vi "Request Config Info.vi"(8 "error in (no error)":errorcluster, 11 "Config Monitor Module in":refnum<class "Config Monitor Module.lvclass">) -> (0 "error out":errorcluster, 3 "Config Monitor Module out":refnum<class "Config Monitor Module.lvclass">)   [LabVIEW 2020, in "VolatusGUI.lvlib" / "Config Monitor Module.lvclass"]
uses:
  Config Monitor Module.lvclass
  C:/dev/lv20CE/relink/lv-volatus/Volatus/Module/Module.lvclass
  System Config Identity/System Config Identity.lvclass
  C:/dev/lv20CE/relink/lv-volatus/Volatus/Identity/Identity.lvclass
  ConfigInfoValue/ConfigInfoValue.lvclass
  Module/Module.lvclass/Module.ctl
  Config Monitor Module.lvclass/Config Monitor Module.ctl
  Module/Module.lvclass
  VolatusAPI/VolatusAPI.lvclass
  MessageQ/MessageQ.lvclass
  C:/dev/lv20CE/relink/lv-volatus/Volatus/Config Alert Module/Config Monitor Module.lvclass
  C:/dev/lv20CE/relink/lv-volatus/Volatus/System Config Identity/System Config Identity.lvclass
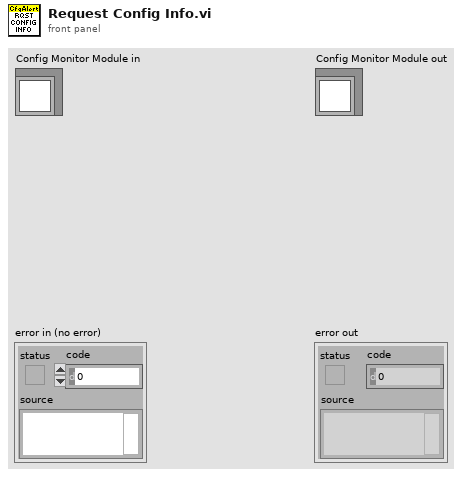
[diagram p1: front panel]
types:
  T1 = typedef "Volatus.lvlib/Config Info.ctl" = cluster{"System":string, "Cluster":string, "Node":string, "Path":path, "Version":string, "Hash":string}
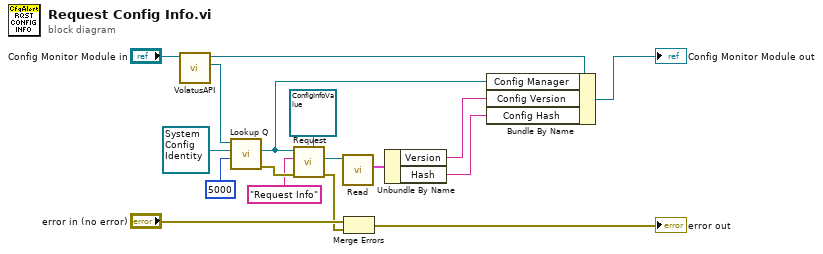
[diagram p0: block diagram]
diagram:
  n1 = call "VolatusAPI.vi"("Module in"="Config Monitor Module in") -> ("VolatusAPI"=w13:refnum<class "VolatusAPI.lvclass">, "Module out"=w14:refnum<class "Config Monitor Module.lvclass">)  [unwired: 9 in]
  n2 = call "Lookup Q.vi"("Timeout ms (0)"=5000, "Identity"=refnum<class "System Config Identity.lvclass"> refnum ("Volatus:System Config Identity.lvclass"), "VolatusAPI in"=w13) -> ("error out"=w17:errorcluster, "MessageQ"=w1:refnum<class "MessageQ.lvclass">)  [unwired: 6 in, 1 out]
  n3 = call "Request.vi"("Response Type (None)"=refnum<class "ConfigInfoValue.lvclass"> refnum ("Volatus:ConfigInfoValue.lvclass"), "error in (no error)"=w17, "ID"="Request Info", "MessageQ in"=w1) -> ("error out"=w2:errorcluster, "Response"=w8:refnum<class "ConfigInfoValue.lvclass">)  [unwired: 5 in, 1 out]
  n4 = call "Read.vi"("ConfigInfoValue in"=w8) -> ("Config Info"=w6:T1)  [unwired: 10 in]
  n5 = Merge Errors("error in (no error)", w2) -> (→"error out":errorcluster)
  n6 = Unbundle By Name(w6) -> ("Version"=w5:string, "Hash"=w4:string)
  n7 = Bundle By Name(cluster=w14, "Config Manager"=w1, "Config Version"=w5, "Config Hash"=w4) -> (→"Config Monitor Module out":refnum<class "Config Monitor Module.lvclass">)
